vi "ADC_GetImmediate.vi"(8 "error in (no error)":errorcluster, 10 "Channel":u32, 11 "DeviceIndex":u32 format="%08x") -> (0 "error out":errorcluster, 3 "pBuf":u32)   [LabVIEW 2012]
doc: "unsigned long ADC_GetImmediate(\nunsigned long DeviceIndex - number from 0-31 indicating from which device you wish to simply\nget data\nunsigned long Channel - number from 0-15 indicating an A/D channel on the device\nunsigned short *pBuf - a pointer to a variable to receive the single A/D sample\n)\nThis function is designed for simplicity. It doesn’t use any of the intermediate features of the\nboard, like calibration or oversampling or even timing, much less any of the advanced features. It\ndoes use the channel’s selected range and single-ended setting, though the defaults are often fine."
uses:
  Windows/System32/AIOUSB.dll
panel:
  out "return type":u32
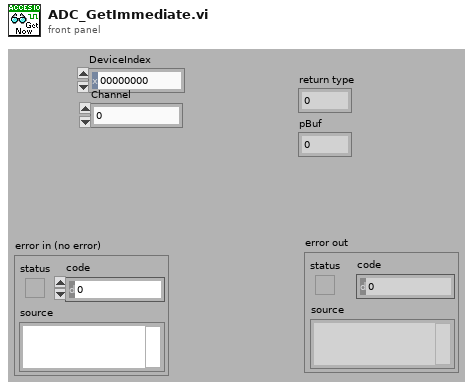
[diagram p1: front panel]
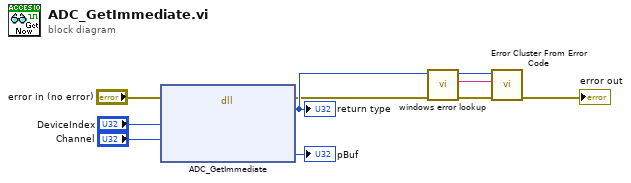
[diagram p0: block diagram]
diagram:
  n1 = dll-call lib="C:/Windows/System32/AIOUSB.dll" fn="ADC_GetImmediate"(error in="error in (no error)", "DeviceIndex"="DeviceIndex", "Channel"="Channel") -> (error out=w1:errorcluster, "return type"=w2:u32, "pBuf"=→"pBuf":u32)  [unwired: 5 in, 1 out]
  "return type" <- w2
  n2 = call "windows error lookup.vi"("error in (no error)"=w1, "Error Code"=w2) -> ("error out"=w4:errorcluster, "error message (\"\")"=w3:string)  [unwired: 8 in]
  n3 = call <vilib>:"Error Cluster From Error Code.vi"("error in (no error)"=w4, "error message (\"\")"=w3, "error code (0)"=w2) -> ("error out"=→"error out":errorcluster)  [unwired: 6 in]
